vi "CCDsetupGLOBAL.vi"() -> ()   [LabVIEW 2020]
panel:
  in  "CCD-ExpTime":dbl=0.2 format="%.2f"
  in  "CCD GPIBadr":i16
  out "CCD-ExpTimeStr":string
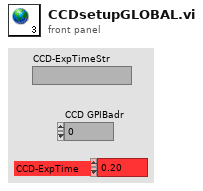
[diagram p1: front panel]
diagram:
